vi "SendMessageToLog2.vi"(7 "Log and view ?":T3, 8 "error in (no error)":errorcluster, 11 "Message":T1) -> (0 "error out":errorcluster)   [LabVIEW 2011]
uses:
  Ctrls/enumLogAndView.ctl
  030 - EVENTS/03 - ToMessageHandlerProcess/ToMessageHandlerEvent.ctl
  030 - EVENTS/03 - ToMessageHandlerProcess/enumMessageCriticity.ctl
  030 - EVENTS/EnumFgvEventCommand.ctl
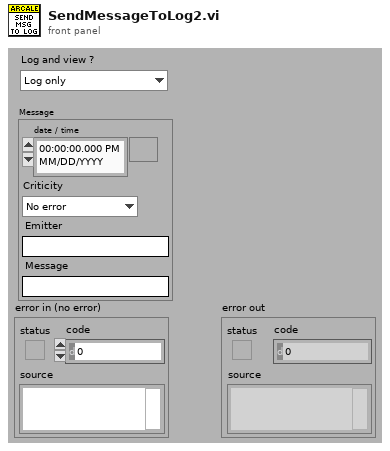
[diagram p1: front panel]
types:
  T1 = typedef "ToMessageHandlerEvent.ctl" = cluster{"date / time":timestamp, "Criticity":T2, "Emitter":string, "Message":string}
  T2 = typedef "enumMessageCriticity.ctl" = enum16{"No error", "Info", "Warning", "Error", "Fatal error"}
  T3 = typedef "enumLogAndView.ctl" = enum16{"Log only", "Log and view"}
  T4 = typedef "EnumFgvEventCommand.ctl" = enum16{"Setup", "Cleanup", "Get"}
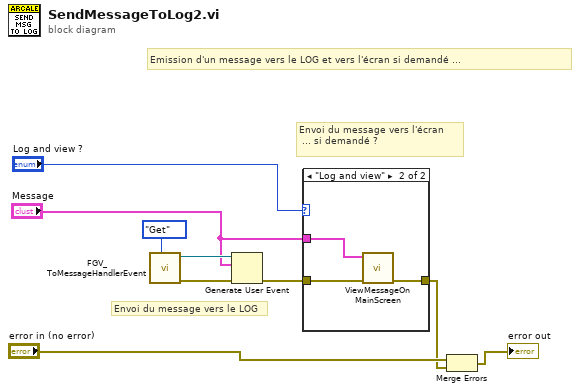
[diagram p0: block diagram]
diagram:
  # "Envoi du message vers l'écran\n ... si demandé ?"
  # "Envoi du message vers le LOG"
  # "Emission d'un message vers le LOG et vers l'écran si demandé ..."
  n1 = call "FGV_ToMessageHandlerEvent.vi"("Command"=EnumFgvEventCommand."Get") -> ("error out"=w8:errorcluster, "To message handler event"=w7:refnum<user-event>)  [unwired: 9 in]
  n2 = Generate User Event(user event=w7, event data cluster="Message", error in=w8) -> (error out=w6:errorcluster)  [unwired: 1 out]
  n3 = case shown="\"Log and view\"" "Log and view ?" {
    tunnel: w6 -> [w10 w13]
    tunnel: [w10 w12] -> w3
    tunnel: "Message" -> [_ w11]
    frame "Log only", Default {
    }
    frame "Log and view" {
      n4 = call "ViewMessageOnMainScreen.vi"("error in (no error)"=w13, "Message"=w11) -> ("error out"=w12:errorcluster)  [unwired: 9 in]
    }
  }
  n5 = Merge Errors("error in (no error)", w3) -> (→"error out":errorcluster)
